vi "Gyro Reset.vi"() -> (0 "Done":bool)   [LabVIEW 2016]
uses:
  Robot Values.vi
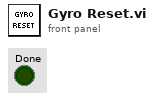
[diagram p1: front panel]
types:
  T1 = typedef "Robot Values.ctl" = cluster{"Robot Drive":cluster{"Left Motor Power":dbl, "Right Motor Power":dbl, "Left Encoder Value":dbl, "Right Encoder Value":dbl, "High Gear?":bool, "PTO?":bool}, "Sensors":cluster{"Gyro Angle":u16, "Recalibrate Gyro":bool, "Reset Gyro":bool}, "Shooter":cluster{"Prep Wheels":bool, "Shoot":bool, "Left Shooter Wheel Speed":dbl, "Wheels Moving":bool, "Shooter Prepped":bool, "Shooter RPS SP":dbl, "Shooting?":bool, "Left Shooter Wheel Power":dbl, "Right Shooter Wheel Power":dbl, "Acquisition Conveyor Power":dbl, "Hopper Beater Bar Power":dbl, "Filtered Left Shooter Speed":dbl, "Acquisition Motor Power":dbl}, "Robot States":cluster{"Drive mode":string, "Alliance":T2, "Position":T3}, "Gear":cluster{"Ejection Active":bool}, "Lights":cluster{"Underglow":string, "License Plate":string, "Hopper":string}}
  T2 = typedef "WPI_DriverStationAllianceInfo.ctl" = enum16{"Red", "Blue", "Invalid"}
  T3 = typedef "WPI_DriverStationPositionInfo.ctl" = enum16{"1", "2", "3"}
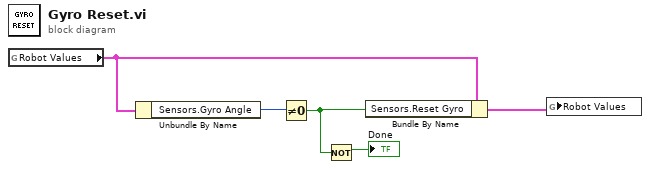
[diagram p0: block diagram]
diagram:
  n1 = global read "Robot Values.vi" "Robot Values"() -> (w5:T1)
  n2 = Unbundle By Name(w5) -> ("Sensors.Gyro Angle"=w4:u16)
  n3 = Not Equal To 0?(x=w4) -> (x != 0?=w3:bool)
  n4 = Not(x=w3) -> (.not. x?=→"Done":bool)
  n5 = Bundle By Name(cluster=w5, "Sensors.Reset Gyro"=w3) -> (w1:T1)
  n6 = global write "Robot Values.vi" "Robot Values"(w1) -> ()
